vi "GUI thinking.vi"() -> ()   [LabVIEW 2020]
panel:
  in  "Sample Average #":dbl
  in  "Number of points #":dbl
  in  "Stop [MHz]":dbl
  in  "Start [MHz]":dbl
  out "Raw graph":dbl[](graph)
  in  "Tab Control":enum32{"Graph", "Calibration"}(tab)
  out "Waveform Graph":dbl[](graph)
  in  "S":bool
  in  "O":bool
  in  "L":bool
  in  "T":bool
  in  "baseline":bool
  in  "Free Run":bool
  in  "Get Data":bool
  in  "Push Settings":bool
  in  "Disconnect":bool
  in  "Stop":bool
  in  "Connect":bool
  # "highest"
  # "lowest"
  # "50C30000"
  # "A1707200"
  # "1354956800"
  # "2708500992"
  # "50kHz"
  # "6Ghz"
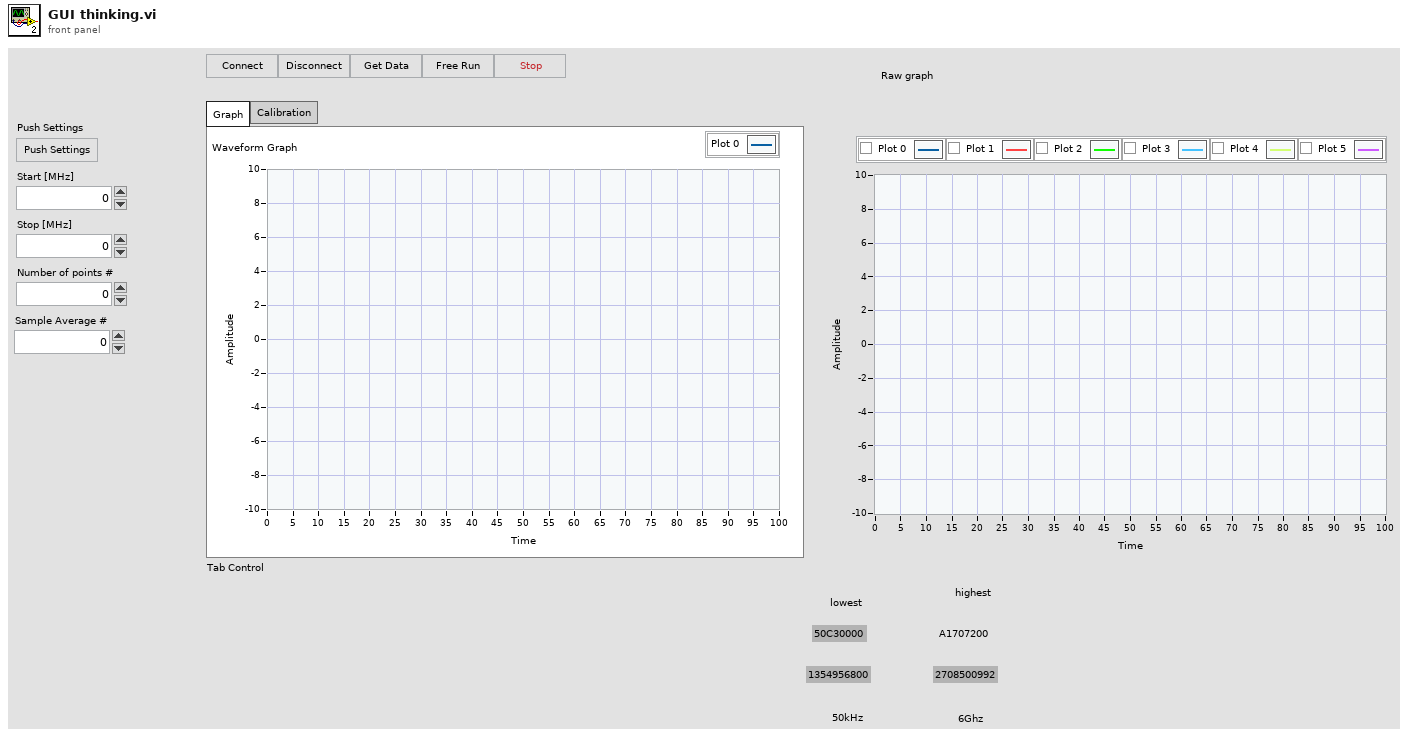
[diagram p1: front panel]
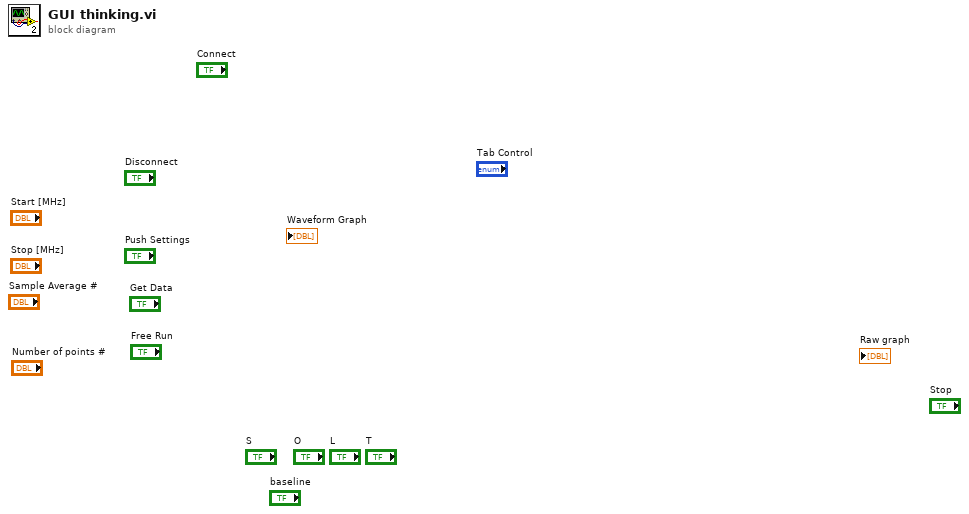
[diagram p0: block diagram]
diagram:
